vi "Yaw Conversion.vi"(11 "Input":dbl) -> (3 "Output":dbl)   [LabVIEW 2016]
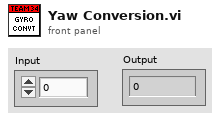
[diagram p1: front panel]
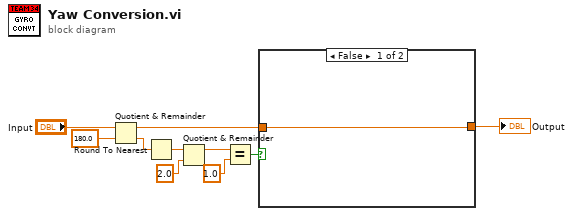
[diagram p0: block diagram]
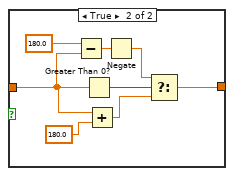
[diagram p2: hidden frame]
diagram:
  n1 = Quotient & Remainder(x="Input", y=180.0) -> (x-y*floor(x/y)=w2:dbl, floor(x/y)=w8:dbl)
  n2 = Round To Nearest(number=w8) -> (nearest integer value=w7:dbl)
  n3 = Quotient & Remainder(x=w7, y=2.0) -> (x-y*floor(x/y)=w5:dbl)  [unwired: 1 out]
  n4 = Equal?(x=w5, y=1.0) -> (x = y?=w3:bool)
  n5 = case shown="False" w3 {
    tunnel: w2 -> [w11 w15]
    tunnel: [w11 w12] -> w1
    frame False {
    }
    frame True {
      n6 = Subtract(x=180.0, y=w15) -> (x-y=w17:dbl)
      n7 = Greater Than 0?(x=w15) -> (x > 0?=w19:bool)
      n8 = Add(x=w15, y=180.0) -> (x+y=w13:dbl)
      n9 = Negate(x=w17) -> (-x=w16:dbl)
      n10 = Select(t=w16, s=w19, f=w13) -> (s? t:f=w12:dbl)
    }
  }
  "Output" <- w1
